vi "Hash File with SHA-256.vi"(8 "error_in":errorcluster, 11 "file_path":path) -> (0 "error_out":errorcluster, 3 "hash":string)   [LabVIEW 2019]
doc: "Calculates the SHA-256 hash for a file on dosc."
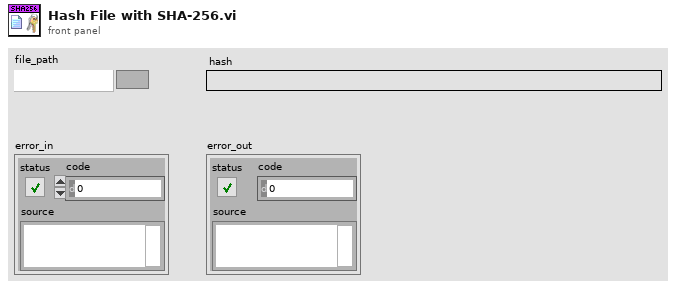
[diagram p1: front panel]
types:
  T1 = enum16{"big-endian, network order", "native, host order", "little-endian"}
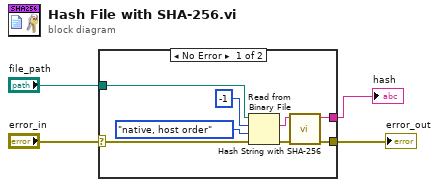
[diagram p0: block diagram]
diagram:
  n1 = case shown="No Error" "error_in" {
    selector: "error_in" -> [w9 w13]
    tunnel: "file_path" -> [w12 _]
    tunnel: [w6 w13] -> w2
    tunnel: [w5 _] -> w1
    frame No Error {
      n2 = Read from Binary File(8:w9, 9:T1."native, host order" ("byte order (0:big-endian, network order)"), 10:-1 ("count (1)"), 11:w12) -> (0:w7:errorcluster, 2:w8:string)  [unwired: 2 in, 2 out]
      n3 = call "Hash String with SHA-256.vi"("error_n"=w7, "string"=w8) -> ("error_out"=w6:errorcluster, "hash"=w5:string)  [unwired: 8 in]
    }
    frame Error {
    }
  }
  "hash" <- w1
  "error_out" <- w2
